vi "BackupOldFolderCreatNewFolder.vi"(8 "error in":errorcluster, 11 "Path":path=path "D:/123/data") -> (0 "error out":errorcluster)   [LabVIEW 2015]
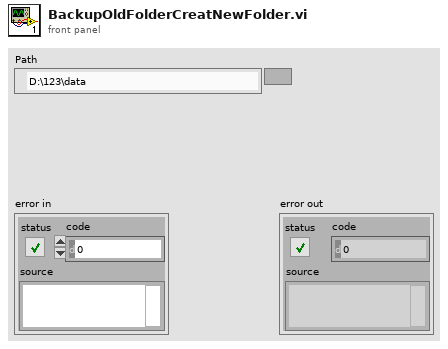
[diagram p1: front panel]
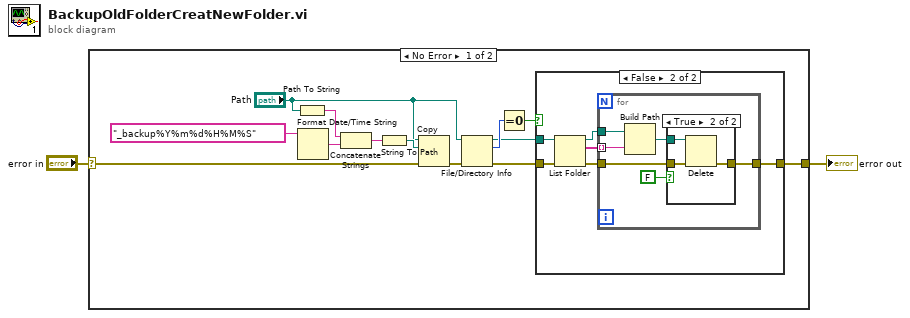
[diagram p0: block diagram]
diagram:
  n1 = case shown="No Error" "error in" {
    selector: "error in" -> [w10 w33]
    tunnel: [w3 w33] -> w1
    frame No Error {
      n2 = Path To String(path="Path") -> (string=w14:string)
      n3 = Format Date/Time String(time format string (%c)="_backup%Y%m%d%H%M%S") -> (date/time string=w13:string)  [unwired: 2 in]
      n4 = Concatenate Strings(w14, w13) -> (w12:string)
      n5 = String To Path(string=w12) -> (path=w11:path)
      n6 = Copy(8:w10, 10:w11, 11:"Path") -> (0:w7:errorcluster)  [unwired: 2 in, 2 out]
      n7 = File/Directory Info(path="Path", error in=w7) -> (path out=w5:path, size=w9:i64, error out=w4:errorcluster)  [unwired: 4 out]
      n8 = Equal To 0?(x=w9) -> (x = 0?=w8:bool)
      n9 = case shown="False" w8 {
        tunnel: w5 -> [_ w20]
        tunnel: w4 -> [w16 w19]
        tunnel: [w16 w17] -> w3
        frame True {
        }
        frame False {
          n10 = List Folder(path=w20, error in=w19) -> (path out=w21:path, filenames=w22:string[], error out=w18:errorcluster)  [unwired: 2 in, 1 out]
          n11 = for {
            tunnel: w22 -> [w27] mode=indexing
            tunnel: w21 -> [w28]
            tunnel: w18 -> [w24]
            tunnel: [w23] -> w17
            n12 = Build Path(base path=w28, name or relative path=w27) -> (appended path=w25:path)
            n13 = case shown="True" FALSE {
              tunnel: w25 -> [_ w32]
              tunnel: w24 -> [w29 w31]
              tunnel: [w29 w30] -> w23
              frame False {
              }
              frame True {
                n14 = Delete(path (use dialog)=w32, error in=w31) -> (error out=w30:errorcluster)  [unwired: 3 in, 2 out]
              }
            }
          }
        }
      }
    }
    frame Error {
    }
  }
  "error out" <- w1
